vi "Find One by ID.vi"(7 "Entity ID":T1, 8 "error in (no error)":errorcluster, 9 "Entity Definition":refnum<class "Type.lvclass">[](array[class]), 10 "Table Name":string, 11 "Database in":refnum<class "SQLite.lvclass">) -> (0 "error out":errorcluster, 2 "Result Row":refnum<class "Result Row.lvclass">, 3 "Database out":refnum<class "SQLite.lvclass">)   [LabVIEW 2022 SP3, in "Conditum SQLite.lvlib" / "SQLite.lvclass"]
uses:
  SQLite.lvclass
  C:/Program Files (x86)/National Instruments/LabVIEW 2022/vi.lib/IlluminatedG/IG Conditum/Conditum/Database Platform/Database Platform.lvclass
  <vilib>/IlluminatedG/IG Conditum/Conditum/Columns/Type/Type.lvclass
  <vilib>/IlluminatedG/IG Conditum/Conditum/Result Row/Result Row.lvclass
  <vilib>/IlluminatedG/IG Conditum/Conditum/Entity ID.ctl
  <vilib>/IlluminatedG/IG Conditum/Conditum/Columns/ID/ID.lvclass
  C:/Program Files (x86)/National Instruments/LabVIEW 2022/vi.lib/IlluminatedG/IG Conditum/Conditum/Columns/Type/Type.lvclass
  <vilib>/IlluminatedG/IG Conditum/Conditum/Columns/ID/ID.lvclass/ID.ctl
  SQLite.lvclass/SQLite.ctl
  <vilib>/IlluminatedG/IG Conditum/Conditum/Columns/Type/Type.lvclass/Type.ctl
  <vilib>/IlluminatedG/IG Conditum/Conditum/Columns/Boolean/Boolean.lvclass
  <vilib>/drjdpowell/SQLite Library/SQL Statement/SQL Statement.lvclass/SQL Statement.ctl
  <vilib>/IlluminatedG/IG Conditum/Conditum/Columns/Boolean/Boolean.lvclass/Boolean.ctl
  <vilib>/IlluminatedG/IG Conditum/Conditum/Columns/Integer/Integer.lvclass
  <vilib>/IlluminatedG/IG Conditum/Conditum/Columns/Integer/Integer.lvclass/Integer.ctl
  <vilib>/IlluminatedG/IG Conditum/Conditum/Columns/Double/Double.lvclass
  <vilib>/IlluminatedG/IG Conditum/Conditum/Columns/Timestamp/Timestamp.lvclass
  <vilib>/IlluminatedG/IG Conditum/Conditum/Columns/Timestamp/Timestamp.lvclass/Timestamp.ctl
  <vilib>/IlluminatedG/IG Conditum/Conditum/Columns/String/String.lvclass
  <vilib>/IlluminatedG/IG Conditum/Conditum/Columns/String/String.lvclass/String.ctl
  <vilib>/drjdpowell/SQLite Library/SQL Statement/Column I64.vi
  <vilib>/drjdpowell/SQLite Library/SQL Statement/Column DBL.vi
  <vilib>/IlluminatedG/IG Conditum/Conditum/Columns/Type/Clear NULL.vi
  <vilib>/drjdpowell/SQLite Library/SQL Statement/Column Type.vi
  <vilib>/drjdpowell/SQLite Library/SQL Statement/Column String.vi
  <vilib>/IlluminatedG/IG Conditum/Conditum/Result Row/Create.vi
  <vilib>/drjdpowell/SQLite Library/SQL Connection/Connection.lvclass
  <vilib>/drjdpowell/SQLite Library/SQL Statement/SQL Statement.lvclass
  <vilib>/IlluminatedG/IG Conditum/Conditum/Database Platform/Database Platform.lvclass
  C:/Program Files (x86)/National Instruments/LabVIEW 2022/vi.lib/IlluminatedG/IG Conditum/Conditum/Columns/Boolean/Boolean.lvclass
  C:/Program Files (x86)/National Instruments/LabVIEW 2022/vi.lib/IlluminatedG/IG Conditum/Conditum/Columns/Integer/Integer.lvclass
  C:/Program Files (x86)/National Instruments/LabVIEW 2022/vi.lib/IlluminatedG/IG Conditum/Conditum/Columns/Double/Double.lvclass
  C:/Program Files (x86)/National Instruments/LabVIEW 2022/vi.lib/IlluminatedG/IG Conditum/Conditum/Columns/Timestamp/Timestamp.lvclass
  C:/Program Files (x86)/National Instruments/LabVIEW 2022/vi.lib/IlluminatedG/IG Conditum/Conditum/Columns/String/String.lvclass
  C:/Program Files (x86)/National Instruments/LabVIEW 2022/vi.lib/IlluminatedG/IG Conditum/Conditum/Columns/ID/ID.lvclass
  C:/dev/lv/illuminated-g/lv-conditum-sqlite/Conditum SQLite/SQLite/SQLite.lvclass
  <vilib>/IlluminatedG/IG Conditum/Conditum/Conditum.lvlib
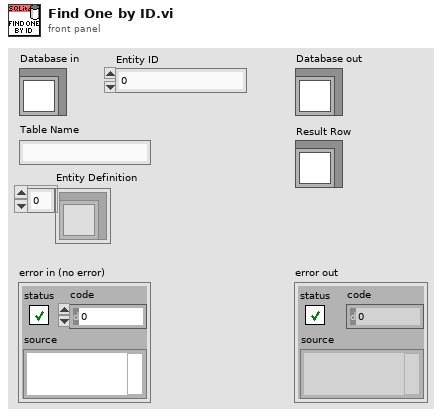
[diagram p1: front panel]
types:
  T1 = typedef "Conditum.lvlib/Entity ID.ctl" = i64
  T2 = typedef "Conditum.lvlib/LabVIEW Type.ctl" = enum16{"None", "ID", "Boolean", "Integer", "Double", "Timestamp", "String", "Text", "Entity"}
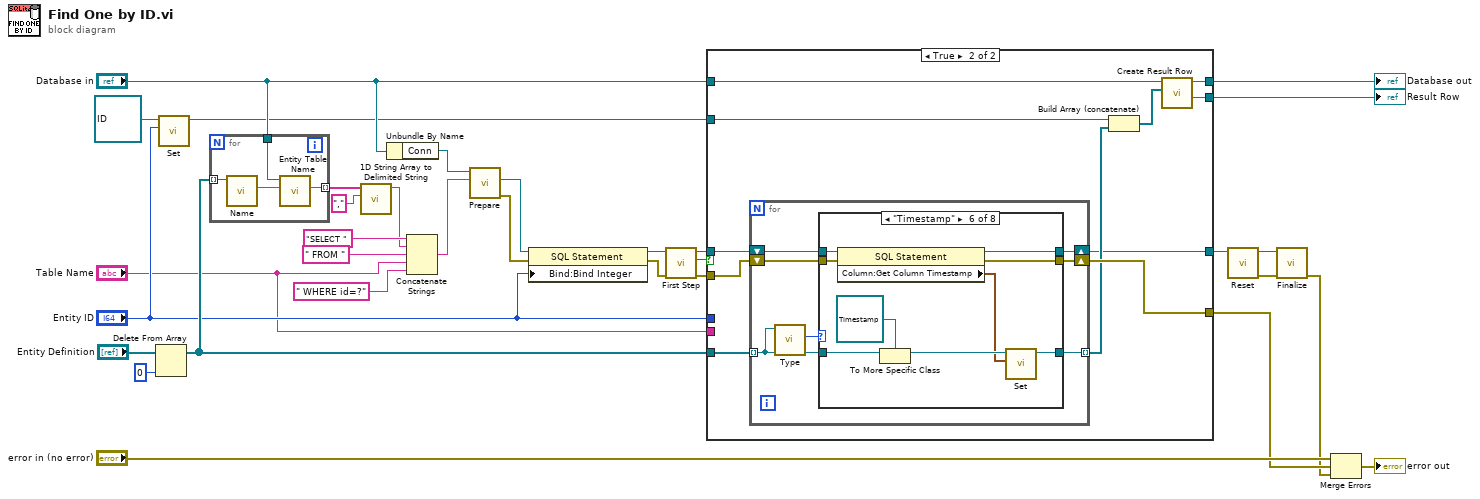
[diagram p0: block diagram]
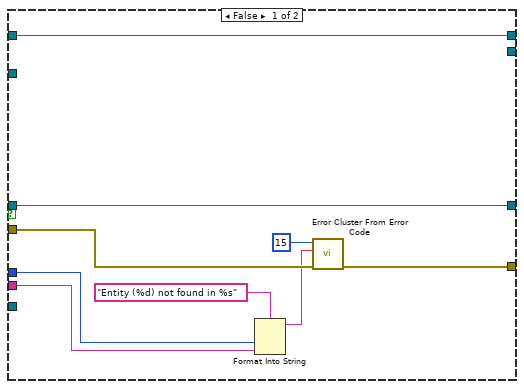
[diagram p2: hidden frame]
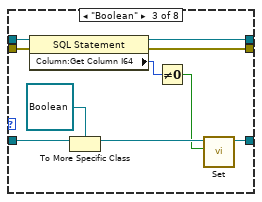
[diagram p5: hidden frame]
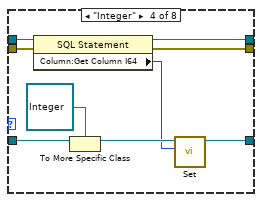
[diagram p6: hidden frame]
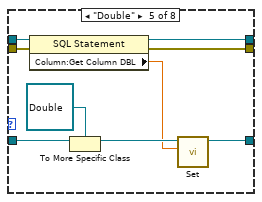
[diagram p7: hidden frame]
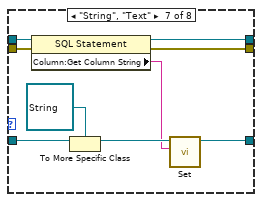
[diagram p8: hidden frame]
diagram:
  n1 = Delete From Array(array="Entity Definition", index=0) -> (array with subset deleted=w24:refnum<class "Type.lvclass">[])  [unwired: 1 in, 1 out]
  n2 = call <vilib>:"Set.vi"("Entity ID"="Entity ID", "ID in"=refnum<class "ID.lvclass"> refnum) -> ("ID out"=w19:refnum<class "ID.lvclass">)  [unwired: 9 in]
  n3 = for {
    tunnel: w24 -> [w36] mode=indexing
    tunnel: [w34] -> w31 mode=indexing
    tunnel: "Database in" -> [w33]
    n4 = call <vilib>:"Name.vi"("Type in"=w36) -> ("Table Name"=w35:string)  [unwired: 10 in]
    n5 = call-dynamic "Entity Table Name.vi"("Entity Name"=w35, "Database in"=w33) -> ("Table Name"=w34:string)  [unwired: 9 in]
  }
  n6 = call <vilib>:"1D String Array to Delimited String.vi"("delimiter"=",", "string array"=w31) -> ("delimited string"=w28:string)  [unwired: 9 in]
  n7 = Unbundle By Name("Database in") -> ("Conn"=w32:refnum<class "Connection.lvclass">)
  n8 = Concatenate Strings("SELECT ", w28, " FROM ", "Table Name", " WHERE id=?") -> (w25:string)
  n9 = call <vilib>:"Prepare.vi"("SQL"=w25, "SQLite Connection in"=w32) -> ("error out"=w13:errorcluster, "SQL Statement"=w14:refnum<class "SQL Statement.lvclass">)  [unwired: 5 in, 3 out]
  n10 = property class="SQL Statement"(reference=w14, error in=w13, "Bind:Bind Integer"="Entity ID") -> (reference out=w12:refnum<class "SQL Statement.lvclass">, error out=w11:errorcluster)
  n11 = call <vilib>:"First Step.vi"("error in (no error)"=w11, "SQL Statement in"=w12) -> ("error out"=w9:errorcluster, "Row returned"=w8:bool, "SQL Statement"=w10:refnum<class "SQL Statement.lvclass">)  [unwired: 7 in]
  n12 = case shown="True" w8 {
    tunnel: [w45 w56] -> w7
    tunnel: w24 -> [_ w55]
    tunnel: "Database in" -> [w41 w54]
    tunnel: [w41 w53] -> w21
    tunnel: w19 -> [_ w52]
    tunnel: [_ w49] -> w18
    tunnel: w10 -> [w43 w48]
    tunnel: w9 -> [w42 w47]
    tunnel: [w43 w46] -> w6
    tunnel: "Entity ID" -> [w39 _]
    tunnel: "Table Name" -> [w38 _]
    frame False {
      n13 = Format Into String(format string="Entity (%d) not found in %s", w39, w38) -> (resulting string=w37:string)  [unwired: 2 in, 1 out]
      n14 = call <vilib>:"Error Cluster From Error Code.vi"("error in (no error)"=w42, "error message (\"\")"=w37, "error code (0)"=15) -> ("error out"=w45:errorcluster)  [unwired: 6 in]
    }
    frame True {
      n15 = for {
        shift-right: [w59] -> w46
        shift-left: w48 -> [w63]
        tunnel: w55 -> [w60] mode=indexing
        tunnel: [w57] -> w51 mode=indexing
        shift-right: [w58] -> w56
        shift-left: w47 -> [w62]
        n16 = call <vilib>:"Type.vi"("Type in"=w60) -> ("Type"=w61:T2)  [unwired: 10 in]
        n17 = case shown="\"Timestamp\"" w61 {
          tunnel: w63 -> [w65 w67 w75 w84 w93 w102 w111 w115]
          tunnel: w62 -> [w64 w66 w74 w83 w92 w101 w110 w114]
          tunnel: w60 -> [_ _ w77 w86 w95 w104 w113 _]
          tunnel: [w65 w67 w73 w82 w91 w100 w109 w115] -> w59
          tunnel: [w64 w66 w72 w81 w90 w99 w108 w114] -> w58
          tunnel: [_ _ w68 w78 w87 w97 w105 _] -> w57
          frame "None", Default {
            # "#ERROR"
          }
          frame "ID" {
            # "#ERROR"
          }
          frame "Boolean" {
            n18 = property class="SQL Statement"(reference=w75, error in=w74) -> (reference out=w73:refnum<class "SQL Statement.lvclass">, error out=w72:errorcluster, "Column:Get Column I64"=w71:i64)
            n19 = To More Specific Class(target class=refnum<class "Boolean.lvclass"> refnum ("Conditum:Columns:Boolean.lvclass"), reference=w77) -> (specific class reference=w70:refnum<class "Boolean.lvclass">)  [unwired: 1 in, 1 out]
            n20 = Not Equal To 0?(x=w71) -> (x != 0?=w69:bool)
            n21 = call <vilib>:"Set.vi"("Value"=w69, "Boolean in"=w70) -> ("Boolean out"=w68:refnum<class "Boolean.lvclass">)  [unwired: 9 in]
          }
          frame "Integer" {
            n22 = property class="SQL Statement"(reference=w84, error in=w83) -> (reference out=w82:refnum<class "SQL Statement.lvclass">, error out=w81:errorcluster, "Column:Get Column I64"=w79:i64)
            n23 = To More Specific Class(target class=refnum<class "Integer.lvclass"> refnum ("Conditum:Columns:Integer.lvclass"), reference=w86) -> (specific class reference=w80:refnum<class "Integer.lvclass">)  [unwired: 1 in, 1 out]
            n24 = call <vilib>:"Set.vi"("Value"=w79, "Integer in"=w80) -> ("Integer out"=w78:refnum<class "Integer.lvclass">)  [unwired: 9 in]
          }
          frame "Double" {
            n25 = property class="SQL Statement"(reference=w93, error in=w92) -> (reference out=w91:refnum<class "SQL Statement.lvclass">, error out=w90:errorcluster, "Column:Get Column DBL"=w88:dbl)
            n26 = To More Specific Class(target class=refnum<class "Double.lvclass"> refnum ("Conditum:Columns:Double.lvclass"), reference=w95) -> (specific class reference=w89:refnum<class "Double.lvclass">)  [unwired: 1 in, 1 out]
            n27 = call <vilib>:"Set.vi"("Value"=w88, "Double in"=w89) -> ("Double out"=w87:refnum<class "Double.lvclass">)  [unwired: 9 in]
          }
          frame "Timestamp" {
            n28 = property class="SQL Statement"(reference=w102, error in=w101) -> (reference out=w100:refnum<class "SQL Statement.lvclass">, error out=w99:errorcluster, "Column:Get Column Timestamp"=w96:timestamp)
            n29 = To More Specific Class(target class=refnum<class "Timestamp.lvclass"> refnum ("Conditum:Columns:Timestamp.lvclass"), reference=w104) -> (specific class reference=w98:refnum<class "Timestamp.lvclass">)  [unwired: 1 in, 1 out]
            n30 = call <vilib>:"Set.vi"("Time Stamp"=w96, "DateTime in"=w98) -> ("DateTime out"=w97:refnum<class "Timestamp.lvclass">)  [unwired: 9 in]
          }
          frame "String", "Text" {
            n31 = property class="SQL Statement"(reference=w111, error in=w110) -> (reference out=w109:refnum<class "SQL Statement.lvclass">, error out=w108:errorcluster, "Column:Get Column String"=w106:string)
            n32 = To More Specific Class(target class=refnum<class "String.lvclass"> refnum ("Conditum:Columns:String.lvclass"), reference=w113) -> (specific class reference=w107:refnum<class "String.lvclass">)  [unwired: 1 in, 1 out]
            n33 = call <vilib>:"Set.vi"("Value"=w106, "String in"=w107) -> ("String out"=w105:refnum<class "String.lvclass">)  [unwired: 9 in]
          }
          frame "Entity" {
            # "#TODO\nRelation update"
          }
        }
      }
      n34 = Build Array (concatenate)(w52, w51) -> (w50:refnum<class "Type.lvclass">[])
      n35 = call <vilib>:"Create Result Row.vi"("Values"=w50, "Database in"=w54) -> ("Result"=w49:refnum<class "Result Row.lvclass">, "Database out"=w53:refnum<class "SQLite.lvclass">)  [unwired: 8 in]
    }
  }
  "Database out" <- w21
  "Result Row" <- w18
  n36 = call <vilib>:"Reset.vi"("SQL Statement in"=w6) -> ("error out"=w4:errorcluster, "SQL Statement"=w5:refnum<class "SQL Statement.lvclass">)  [unwired: 9 in]
  n37 = call <vilib>:"Finalize.vi"("error in (no error)"=w4, "SQL Statement in"=w5) -> ("error out"=w3:errorcluster)  [unwired: 9 in]
  n38 = Merge Errors("error in (no error)", w7, w3) -> (→"error out":errorcluster)
